vi "BooleanFG.vi"(1 "Read Or Write":enum16{"Read", "Write"}(ring)=enum."Write", 2 "Bool In":bool) -> (0 "Bool Out":bool)   [LabVIEW 2016]
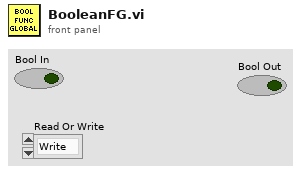
[diagram p1: front panel]
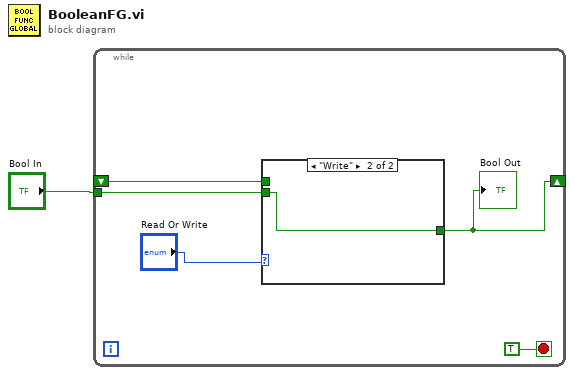
[diagram p0: block diagram]
diagram:
  n1 = while {
    shift-right: [w2] -> _
    shift-left: _ -> [w5]
    tunnel: "Bool In" -> [w3]
    stop <- TRUE stop-if-true
    n2 = case shown="\"Write\"" "Read Or Write" {
      tunnel: [w7 w8] -> w2
      tunnel: w5 -> [w7 _]
      tunnel: w3 -> [_ w8]
      frame "Read", Default {
      }
      frame "Write" {
      }
    }
    "Bool Out" <- w2
  }
